vi "FPGA Toggle.vi"(8 "error in (no error)":errorcluster, 11 "fpgaCommand":u8) -> (0 "error out":errorcluster, 3 "function return":i32)   [LabVIEW 2013, in "Stats32.lvlib"]
doc: "LIBRARY_API int FPGA_Toggle(unsigned char fpgaCommand);"
uses:
  Stats32.lvlib
  Stats/Release/Win32/Stats32.dll
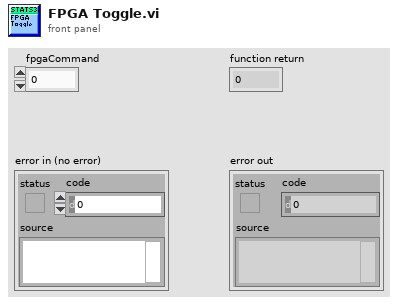
[diagram p1: front panel]
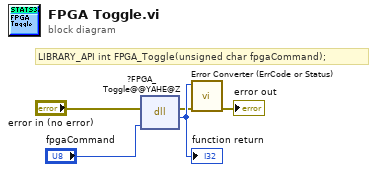
[diagram p0: block diagram]
diagram:
  # "LIBRARY_API int FPGA_Toggle(unsigned char fpgaCommand);"
  n1 = dll-call lib="C:/Programming/Stats/Stats/Release/Win32/Stats32.*" fn="?FPGA_Toggle@@YAHE@Z"(error in="error in (no error)", "fpgaCommand"="fpgaCommand") -> (error out=w2:errorcluster, w5:i32)  [unwired: 3 in, 1 out]
  "function return" <- w5
  n2 = call "Error Converter (ErrCode or Status).vi"("error in (no error)"=w2, "error code"=w5) -> ("error out"=→"error out":errorcluster)  [unwired: 9 in]
